vi "Set Index.vi"(8 "error in":errorcluster, 10 "Index":u16, 11 "OD Subentry in":refnum<class "OD Subentry.lvclass">) -> (0 "error out":errorcluster, 3 "OD Subentry out":refnum<class "OD Subentry.lvclass">)   [LabVIEW 2024, in "EDS.lvlib" / "OD Subentry.lvclass"]
uses:
  OD Subentry.lvclass
  OD Subentry.lvclass/OD Subentry.ctl
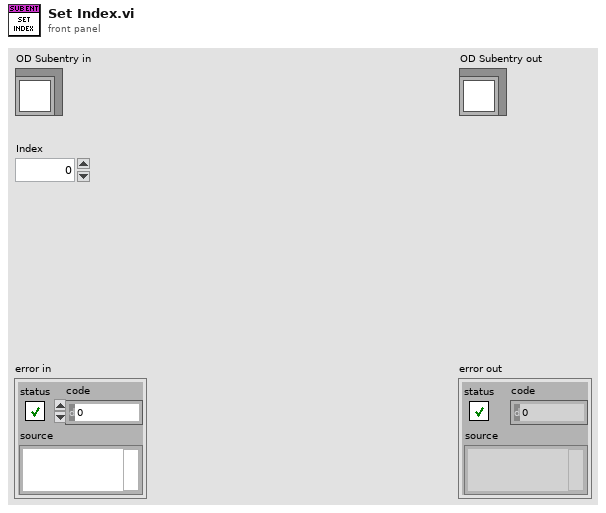
[diagram p1: front panel]
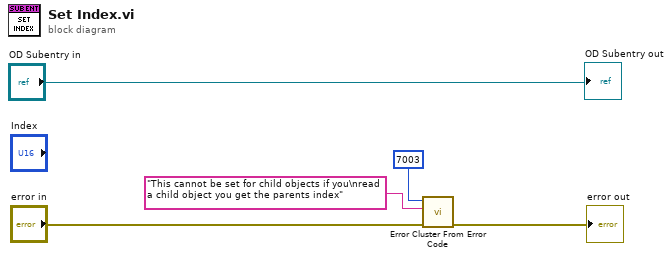
[diagram p0: block diagram]
diagram:
  n1 = call <vilib>:"Error Cluster From Error Code.vi"("error in (no error)"="error in", "error message (\"\")"="This cannot be set for child objects if you\nread a child object you get the parents index" ("error message (\"\")"), "error code (0)"=7003) -> ("error out"=→"error out":errorcluster)  [unwired: 6 in]
  "OD Subentry out" <- "OD Subentry in"
